vi "Shooter Controller.vi"(8 "error in":errorcluster) -> ()   [LabVIEW 2020]
doc: "This VI executes continuously carrying out the current operation and responding to updates or new operations. It will often contain the timing or control code that is difficult to place directly in TeleOp. This VI generally opens all sensors and motors and isolates the rest of the robot code from knowing how the operations are carried out."
uses:
  <vilib>/Rock Robotics/WPI/Framework/Completion Status.ctl
  Shooter Setpoints.ctl
  Shooter Operations.ctl
  <vilib>/Rock Robotics/WPI/SafetyOutput/WPI_SafetyOutputConfigMenu.ctl
  <vilib>/Rock Robotics/Network Tables/NT Write Number.vi
panel:
  in  "Interactive Values":T1
  out "Current\nCmd":string
  in  "Buttons":cluster{"Execute Cmd":bool, "Abort Cmd":bool}
  out "Command Timing":cluster{"Start Time (ms)":u32, "Iterations":i32}
  out "Status":T3
  # "Tip: It may be helpful to observe inputs and sensor values.\nYou may also want to display tuning or debugging controls."
  # "Interactive Command: You may fill in the settings for a command\nand schedule it with the Execute button. You can observe and abort\nany command while fine tuning the code for the controller."
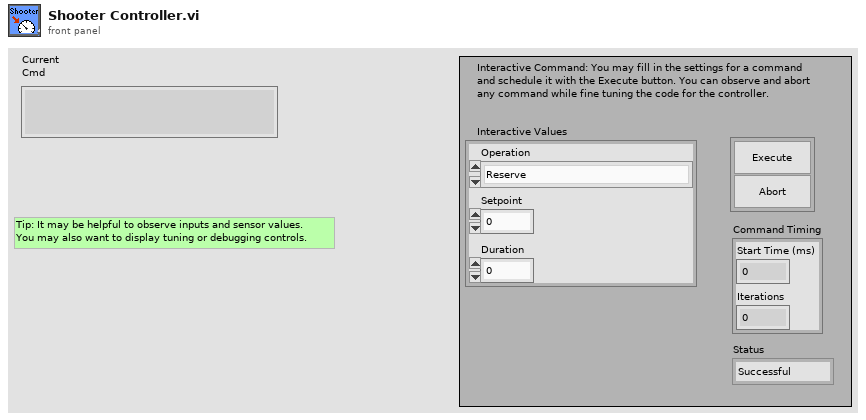
[diagram p1: front panel]
types:
  T1 = typedef "Shooter Setpoints.ctl" = cluster{"Operation":T2, "Setpoint":dbl, "Duration":dbl}
  T2 = typedef "Shooter Operations.ctl" = enum16{"Reserve", "Read Current", "Immediate", "with Duration", "Stop"}
  T3 = typedef "Completion Status.ctl" = enum16{"Successful", "Aborted", "Incomplete"}
  T4 = typedef "WPI_SafetyOutputConfigMenu.ctl" = enum16{"Enable", "Disable"}
  T5 = typedef "WPI_MotorControlDeviceRef.ctl" = cluster{"DeviceStatus":errorcluster, "Type":T6, "PWM":cluster{"PWM Channel":T7, "DeadBand":T8}, "CAN":cluster{"Device Number":u8, "SetOutput VI Ref":variant, "GetOutput VI Ref":variant, "Enable VI Ref":variant, "Disable VI Ref":variant, "Data":variant}, "Invert":bool, "DIO PWM":cluster{"PWM \"Enable\" Channel":T7, "DIOChannel":T9, "PWM Rate":dbl}}
  T6 = typedef "WPI_MotorControlType.ctl" = enum16{"PWM", "CAN", "DIO PWM"}
  T7 = typedef "FPGA_DIOPWMChannel.ctl" = enum8{"PWM 0", "PWM 1", "PWM 2", "PWM 3", "PWM 4", "PWM 5", "PWM 6", "PWM 7", "PWM 8", "PWM 9", "PWM MXP 0", "PWM MXP 1", "PWM MXP 2", "PWM MXP 3", "PWM MXP 4", "PWM MXP 5", "PWM MXP 6", "PWM MXP 7", "PWM MXP 8", "PWM MXP 9", "Invalid"}
  T8 = typedef "WPI_PWMDeadband.ctl" = cluster{"Name":string, "maxPositivePwm":i32, "minPositivePwm":i32, "centerPwm":i32, "maxNegativePwm":i32, "minNegativePwm":i32, "angularRange":u16}
  T9 = typedef "FPGA_DIOChannel.ctl" = enum8{"DIO 0", "DIO 1", "DIO 2", "DIO 3", "DIO 4", "DIO 5", "DIO 6", "DIO 7", "DIO 8", "DIO 9", "DIO MXP 0", "DIO MXP 1", "DIO MXP 2", "DIO MXP 3", "DIO MXP 4", "DIO MXP 5", "DIO MXP 6", "DIO MXP 7", "DIO MXP 8", "DIO MXP 9", "DIO MXP 10", "DIO MXP 11", "DIO MXP 12", "DIO MXP 13", "DIO MXP 14", "DIO MXP 15", "SPI Port CS1", "SPI Port CS2", "SPI Port CS3", "SPI Port MISO", "SPI Port MOSI", "Invalid"}
  T10 = typedef "Command Status Info.ctl" = cluster{"Name":string, "Status":T3, "notifier out":T11}
  T11 = typedef "Completion Notifier.ctl" = refnum<notifier>
  T12 = cluster{"Current Command":T1, "Command Timing":cluster{"Start Time (ms)":u32, "Iterations":i32}, "Command Arguments":cluster{"Command Info":T10, "Description":string, "Default Command":T1, "queue out":refnum<queue>, "Subsystem Name":string}}
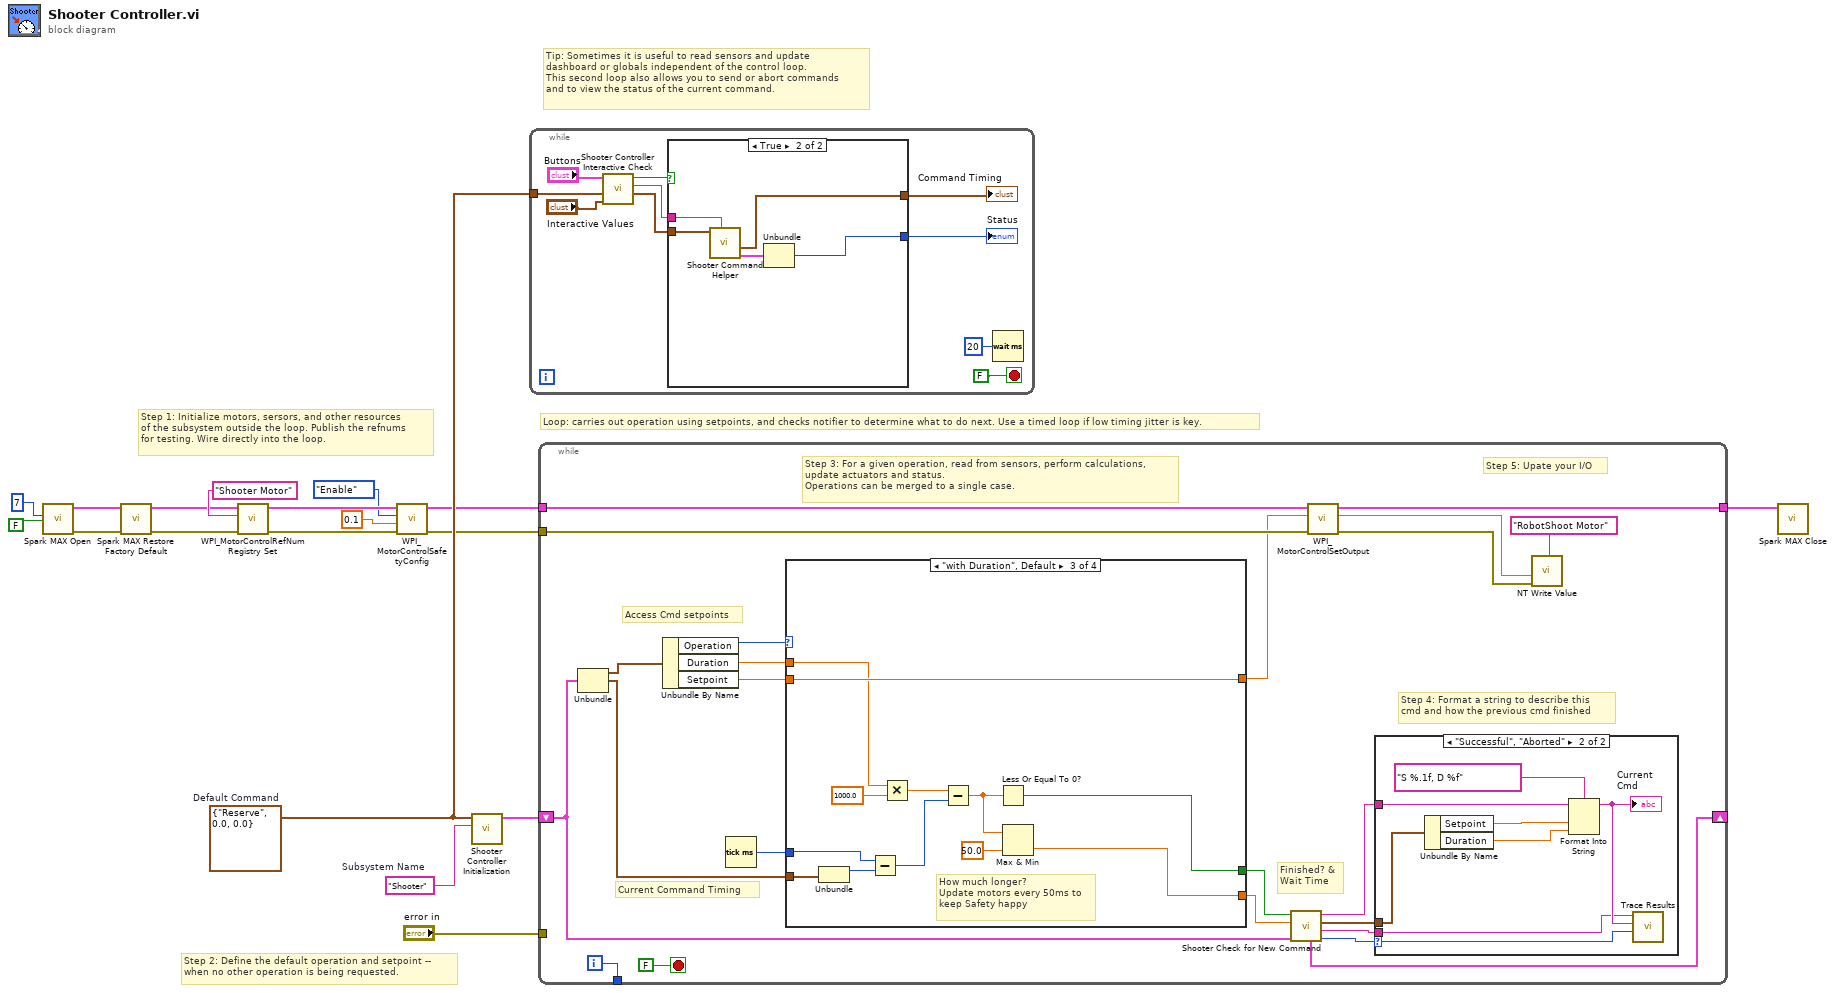
[diagram p0: block diagram]
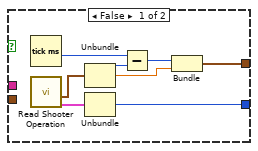
[diagram p2: hidden frame]
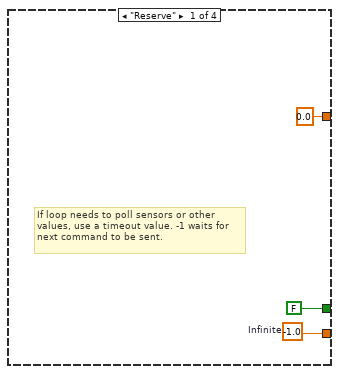
[diagram p4: hidden frame]
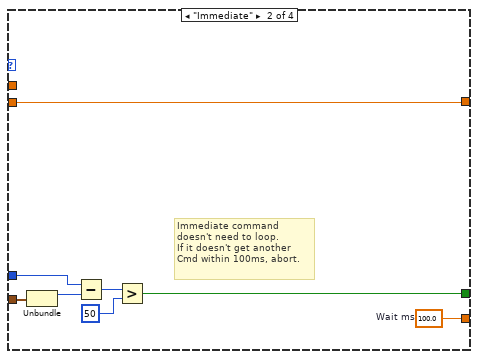
[diagram p5: hidden frame]
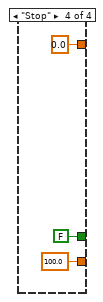
[diagram p6: hidden frame]
diagram:
  w15 = T1 {"Operation"=enum."Reserve", "Setpoint"=0.0, "Duration"=0.0}  # Default Command
  w16 = "Shooter"  # Subsystem Name
  # "Tip: Sometimes it is useful to read sensors and update\ndashboard or globals independent of the control loop.\nThis second loop also allows you to send or abort commands\nand to view the status of the current command."
  # "Step 2: Define the default operation and setpoint --\nwhen no other operation is being requested."
  # "Step 1: Initialize motors, sersors, and other resources\nof the subsystem outside the loop. Publish the refnums\nfor testing. Wire directly into the loop."
  # "Loop: carries out operation using setpoints, and checks notifier to determine what to do next. Use a timed loop if low timing jitter is key."
  n1 = call <vilib>:"Spark MAX Open.vi"("Invert"=FALSE, "Device Number"=u8 7) -> ("error out"=w5:errorcluster, "MotorControlDeviceRef"=w7:T5)  [unwired: 8 in]
  n2 = call <vilib>:"Spark MAX Restore Factory Default.vi"("error in"=w5, "MotorControlDeviceRef"=w7) -> ("error out"=w4:errorcluster, "MotorControlDeviceRef"=w6:T5)  [unwired: 8 in]
  n3 = call <vilib>:"WPI_MotorControlRefNum Registry Set.vi"("error in (no error)"=w4, "refnum name"="Shooter Motor", "MotorControlDevRef"=w6) -> ("error out"=w14:errorcluster, "MotorControlDevRef"=w13:T5)  [unwired: 7 in]
  n4 = call <vilib>:"WPI_MotorControlSafetyConfig.vi"("error in (no error)"=w14, "timeout (s)"=0.1, "mode"=WPI_SafetyOutputConfigMenu."Enable", "MotorControlDevRef"=w13) -> ("error out"=w1:errorcluster, "MotorControlDevRef"=w3:T5)  [unwired: 6 in]
  n5 = call "Shooter Controller Initialization.vi"("Subsystem Name"=w16, "Default Command"=w15) -> ("Current Command"=w17:T12)  [unwired: 9 in]
  n6 = while {
    tunnel: w15 -> [w25]
    stop <- FALSE stop-if-true
    n7 = call "Shooter Controller Interactive Check.vi"("Interactive Command in"="Interactive Values", "Default Command"=w25, "Buttons"="Buttons") -> ("Interactive Command out"=w22:T1, "Trace String"=w23:string, "Schedule"=w24:bool)  [unwired: 6 in]
    n8 = case shown="True" w24 {
      tunnel: [w36 w41] -> w21
      tunnel: w22 -> [_ w39]
      tunnel: [w32 w37] -> w20
      tunnel: w23 -> [_ w40]
      frame False {
        n9 = Tick Count (ms)() -> (millisecond timer value=w31:u32)
        n10 = call "Read Shooter Operation.vi"() -> ("Command Info"=w29:T10, "SubSystem Data"=w30:T1)  [unwired: 9 in, 1 out]
        n11 = Unbundle(w30) -> ("Operation"=w35:T2, "Setpoint"=w33:dbl)  [unwired: 1 out]
        n12 = Unbundle(w29) -> ("Status"=w36:T3)  [unwired: 2 out]
        n13 = Subtract(x=w31, y=w35) -> (x-y=w34:u32)
        n14 = Bundle(w34, "Setpoint"=w33) -> (w32:cluster{u32, "Setpoint":dbl})  [unwired: 1 in]
      }
      frame True {
        n15 = call "Shooter Command Helper.vi"("Description"=w40, "SubSystem Data"=w39) -> ("Command Info Out"=w38:T10, "Command Timing"=w37:cluster{"Start Time (ms)":u32, "Iterations":i32})  [unwired: 7 in, 1 out]
        n16 = Unbundle(w38) -> ("Status"=w41:T3)  [unwired: 2 out]
      }
    }
    "Status" <- w21
    "Command Timing" <- w20
    n17 = Wait (ms)(milliseconds to wait=u32 20) -> ()  [unwired: 1 out]
  }
  n18 = while {
    shift-right: [w56] -> _
    shift-left: w17 -> [w49]
    tunnel: [w63] -> _
    tunnel: "error in" -> [_]
    tunnel: w3 -> [w48]
    tunnel: [w47] -> w2
    tunnel: w1 -> [w46]
    i -> [w63]
    stop <- FALSE stop-if-true
    # "Step 5: Upate your I/O"
    # "Step 4: Format a string to describe this\ncmd and how the previous cmd finished"
    # "Current Command Timing"
    # "Access Cmd setpoints"
    # "Finished? &\nWait Time"
    # "Step 3: For a given operation, read from sensors, perform calculations,\nupdate actuators and status.\nOperations can be merged to a single case."
    n19 = Unbundle(w49) -> ("Current Command"=w62:T1, "Command Timing"=w58:cluster{"Start Time (ms)":u32, "Iterations":i32})  [unwired: 1 out]
    n20 = Unbundle By Name(w62) -> ("Operation"=w61:T2, "Duration"=w60:dbl, "Setpoint"=w57:dbl)
    n21 = Tick Count (ms)() -> (millisecond timer value=w59:u32)
    n22 = case shown="\"with Duration\", Default" w61 {
      tunnel: [w75 w83 w86 100.0 ("Infinite")] -> w54
      tunnel: [FALSE ("ignore previous (F)") w77 w87 FALSE ("ignore previous (F)")] -> w55
      tunnel: w58 -> [_ w79 w89 _]
      tunnel: w60 -> [_ _ w84 _]
      tunnel: w59 -> [_ w78 w88 _]
      tunnel: w57 -> [_ w76 w85 _]
      tunnel: [0.0 ("Setpoint") w76 w85 0.0 ("Setpoint")] -> w45
      frame "Reserve" {
        w75 = -1.0  # Infinite
        # "If loop needs to poll sensors or other\nvalues, use a timeout value. -1 waits for\nnext command to be sent."
      }
      frame "Immediate" {
        w83 = 100.0  # Wait ms
        # "Immediate command\ndoesn't need to loop.\nIf it doesn't get another\nCmd within 100ms, abort."
        n23 = Unbundle(w79) -> ("Start Time (ms)"=w82:u32)  [unwired: 1 out]
        n24 = Subtract(x=w78, y=w82) -> (x-y=w81:u32)
        n25 = Greater?(x=w81, y=u8 50 ("Left Motor")) -> (0:w77:bool)
      }
      frame "with Duration", Default {
        # "How much longer?\nUpdate motors every 50ms to\nkeep Safety happy"
        n26 = Unbundle(w89) -> ("Start Time (ms)"=w94:u32)  [unwired: 1 out]
        n27 = Subtract(x=w88, y=w94) -> (x-y=w92:u32)
        n28 = Multiply(x=w84, y=1000.0) -> (x*y=w93:dbl)
        n29 = Subtract(x=w93, y=w92) -> (x-y=w95:dbl)
        n30 = Less Or Equal To 0?(x=w95) -> (x <= 0?=w87:bool)
        n31 = Max & Min(x=w95, y=50.0) -> (min(x,y)=w86:dbl)  [unwired: 1 out]
      }
      frame "Stop" {
      }
    }
    n32 = call "Shooter Check for New Command.vi"("Current Command"=w49, "Wait time (ms)"=w54, "Finished?"=w55) -> ("Completion"=w50:T3, "Subsystem Name"=w51:string, "Current Command"=w52:T1, "Initial Trace String"=w53:string, "NextCommand"=w56:T12)  [unwired: 4 in]
    n33 = call <vilib>:"WPI_MotorControlSetOutput.vi"("error in (no error)"=w46, "Output"=w45, "MotorControlDevRef"=w48) -> ("error out"=w43:errorcluster, "Motor Output"=w44:dbl, "MotorControlDevRef"=w47:T5)  [unwired: 6 in]
    n34 = case shown="\"Successful\", \"Aborted\"" w50 {
      selector: w50 -> [_ w72]
      tunnel: w53 -> [_ w68]
      tunnel: w52 -> [_ w69]
      tunnel: w51 -> [_ w65]
      frame "Incomplete", Default {
        # "Continuing current command"
      }
      frame "Successful", "Aborted" {
        # "Report and setup for next command"
        n35 = Unbundle By Name(w69) -> ("Setpoint"=w71:dbl, "Duration"=w66:dbl)
        n36 = Format Into String(format string="S %.1f, D %f", initial string=w68, w71, w66) -> (resulting string=w67:string)  [unwired: 1 in, 1 out]
        "Current\nCmd" <- w67
        n37 = call <vilib>:"Trace Results.vi"("Status of previous command"=w72, "Description"=w67, "Subsystem"=w65) -> ()  [unwired: 9 in]
      }
    }
    n38 = call-poly <vilib>:"NT Write Value.vi"("error in"=w43, "Numeric"=w44, "Name"="RobotShoot Motor") -> ()  [unwired: 8 in, 1 out]
  }
  n39 = call <vilib>:"Spark MAX Close.vi"("MotorControlDeviceRef"=w2) -> ()  [unwired: 10 in, 1 out]
